vi "FRCts20_Backend_Event_POST.vi"(8 "error in (no error)":errorcluster, 9 "Duration":u8, 10 "Start Date":timestamp, 11 "Name":string) -> (0 "error out":errorcluster, 1 "Time (ms)":u32, 2 "Status":string, 3 "Event Out":T1, 5 "Success":bool)   [LabVIEW 2013]
uses:
  FRCts20_Backend_API/FRCts20_Backend_API_Command_Event.ctl
  FRCts20_Backend_API/FRCts20_Backend_API.lvlib
  FRCts20_Backend_API/FRCts20_Backend_API_Event.ctl
  FRCts20_Backend_API/FRCts20_Backend_API_Event.vi
  FRCts20_Backend_API/FRCts20_Backend_API_SW.ctl
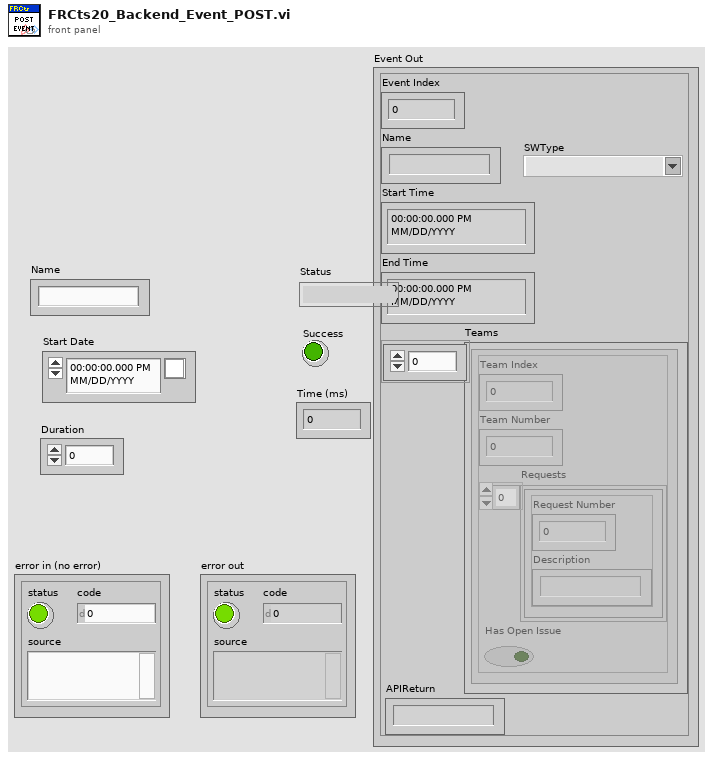
[diagram p1: front panel]
types:
  T1 = typedef "FRCts20_Backend_API.lvlib/FRCts20_Backend_API_Event.ctl" = cluster{"Event Index":u32, "Name":string, "Start Time":timestamp, "End Time":timestamp, "Teams":cluster{"Team Index":u32, "Team Number":u32, "Requests":cluster{"Request Number":u32, "Description":string}[], "Has Open Issue":bool}[], "SWType":T2, "APIReturn":string}
  T2 = typedef "FRCts20_Backend_API.lvlib/FRCts20_Backend_API_SW.ctl" = string
  T3 = typedef "FRCts20_Backend_API.lvlib/FRCts20_Backend_API_Command_Event.ctl" = string
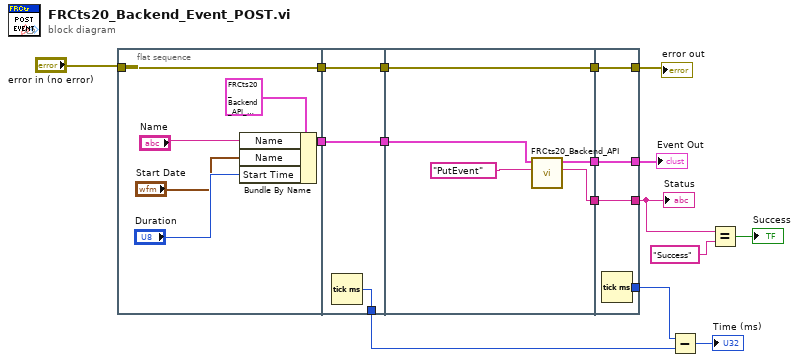
[diagram p0: block diagram]
diagram:
  n1 = flat-sequence {
    tunnel: "error in (no error)" -> [w22]
    tunnel: [w22] -> w16
    tunnel: [w21] -> w15
    tunnel: [w25] -> w3
    tunnel: [w24] -> w14
    tunnel: w16 -> [w24]
    tunnel: [w23] -> w13
    tunnel: w15 -> [w23]
    tunnel: [w30] -> w12
    tunnel: w14 -> [w30]
    tunnel: w13 -> [w28]
    tunnel: [w27] -> w11
    tunnel: [w26] -> w10
    tunnel: [w34] -> w4
    tunnel: [w33] -> w6
    tunnel: w12 -> [w33]
    tunnel: [w32] -> w2
    tunnel: w11 -> [w32]
    tunnel: [w31] -> w1
    tunnel: w10 -> [w31]
    frame #0 {
      n2 = Bundle By Name(cluster=T1 {"Event Index"=0, "Name"="", "Start Time"=timestamp(0 s since 1904-01-01), "End Time"=timestamp(0 s since 1904-01-01), "Teams"=[], "SWType"="", "APIReturn"=""} ("Event In"), "Name"="Name", "Name"="Start Date", "Start Time"="Duration") -> (w21:T1)
    }
    frame #1 {
      n3 = Tick Count (ms)() -> (millisecond timer value=w25:u32)
    }
    frame #2 {
      n4 = call-poly "FRCts20_Backend_API.vi"("Command"=T3 "PutEvent", "Event In"=w28) -> ("Status"=w26:string, "Event Out"=w27:T1)  [unwired: 7 in, 1 out]
    }
    frame #3 {
      n5 = Tick Count (ms)() -> (millisecond timer value=w34:u32)
    }
  }
  n6 = Subtract(x=w4, y=w3) -> (x-y=→"Time (ms)":u32)
  n7 = Equal?(x=w1, y="Success") -> (x = y?=→"Success":bool)
  "Event Out" <- w2
  "Status" <- w1
  "error out" <- w6
